vi "TDTSyn-Initialize.vi"() -> (4 "Settings":T1={"Server IP Address"=4925, "TCP Port"=4925, "Synapse URL"="", "Tank Root"=""}, 15 "error out":errorcluster)   [LabVIEW 2020]
uses:
  TDTSyn-Settings.ctl
  <vilib>/Utility/config.llb/Read Key (String).vi
  <vilib>/Utility/config.llb/Read Key (I32).vi
  <vilib>/Utility/config.llb/NI_LVConfig.lvlib
panel:
  in  "error in (no error)":errorcluster
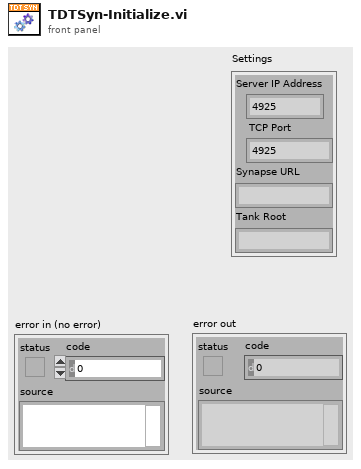
[diagram p1: front panel]
types:
  T1 = typedef "TDTSyn-Settings.ctl" = cluster{"Server IP Address":u32, "TCP Port":u16, "Synapse URL":string, "Tank Root":string}
  T2 = typedef "NI_LVConfig.lvlib/Config Data RefNum.ctl" = refnum<k1>
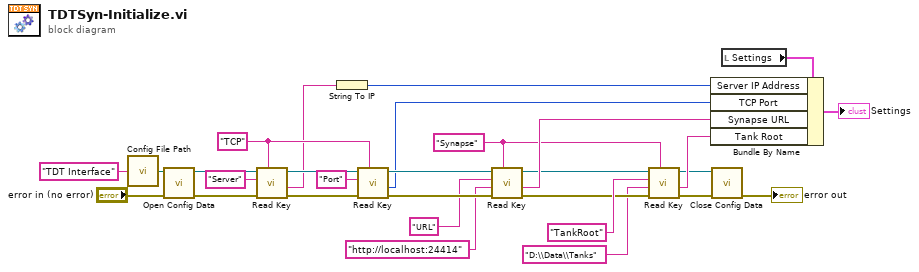
[diagram p0: block diagram]
diagram:
  w7 = "Synapse" ("section")
  w24 = "TCP" ("section")
  n1 = call "Config File Path.vi"("AppName"="TDT Interface") -> ("Default config file name"=w5:path)
  n2 = call <vilib>:"Open Config Data.vi"("error in (no error)"="error in (no error)", "configuration file path"=w5) -> ("error out"=w28:errorcluster, "refnum"=w29:T2)  [unwired: 7 in, 1 out]
  n3 = call-poly <vilib>:"Read Key.vi"("section"=w24, "error in (no error)"=w28, "key"="Server", "refnum"=w29) -> ("error out"=w26:errorcluster, "value"=w22:string, "refnum out"=w25:T2)  [unwired: 4 in, 1 out]
  n4 = String To IP(1:w22) -> (0:w4:u32)
  n5 = call-poly <vilib>:"Read Key.vi"("section"=w24, "error in (no error)"=w26, "key"="Port", "refnum"=w25) -> ("error out"=w17:errorcluster, "value"=w2:i32, "refnum out"=w18:T2)  [unwired: 4 in, 1 out]
  n6 = call-poly <vilib>:"Read Key.vi"("section"=w7, "error in (no error)"=w17, "default value"="http://localhost:24414", "key"="URL", "refnum"=w18) -> ("error out"=w12:errorcluster, "value"=w14:string, "refnum out"=w11:T2)  [unwired: 3 in, 1 out]
  n7 = call-poly <vilib>:"Read Key.vi"("section"=w7, "error in (no error)"=w12, "default value"="D:\\Data\\Tanks" ("key"), "key"="TankRoot", "refnum"=w11) -> ("error out"=w9:errorcluster, "value"=w10:string, "refnum out"=w8:T2)  [unwired: 3 in, 1 out]
  n8 = call <vilib>:"Close Config Data.vi"("error in (no error)"=w9, "refnum"=w8) -> ("error out"=→"error out":errorcluster)  [unwired: 8 in, 1 out]
  n9 = local read "Settings"() -> (w19:T1)
  n10 = Bundle By Name(cluster=w19, "Server IP Address"=w4, "TCP Port"=w2, "Synapse URL"=w14, "Tank Root"=w10) -> (→"Settings":T1)
